vi "SolenoidB.vi"() -> (3 "Thermometer":dbl(slide) scale=140.0..160.0)   [LabVIEW 2018, in "com.Instrument.lvlib"]
uses:
  com.Instrument.lvlib
  global/Solenoid Temp.vi
panel:
  in  "Slide":dbl(slide) scale=140.0..170.0
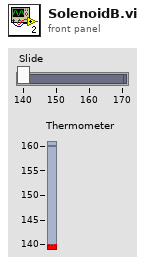
[diagram p1: front panel]
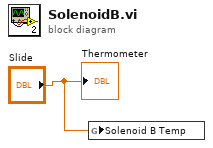
[diagram p0: block diagram]
diagram:
  n1 = global write "Solenoid Temp.vi" "Solenoid B Temp"("Slide") -> ()
  "Thermometer" <- "Slide"
